vi "WCA_GET_SIS_MODE.vi"(0 "Cartridge Band":u32=10, 1 "Slave Node in":cluster{"Address":i16, "Serial Number":i8[]}={"Address"=19, "Serial Number"=[16, 71, 55, 76, 1, 8, 0, -15]} {"Serial Number" format="%.0x"; "Address" format="%.0x"}, 2 "ObjHandle in":u32, 5 "POL":u32, 7 "sb":u32=1, 11 "error in (no error)":errorcluster) -> (4 "ObjHandle out":u32=92930112, 8 "GET_SIS_MODE":u8, 15 "error out":errorcluster)   [LabVIEW 2017]
uses:
  WCA_Global.vi
panel:
  # "Node Address"
  # "Serial Number"
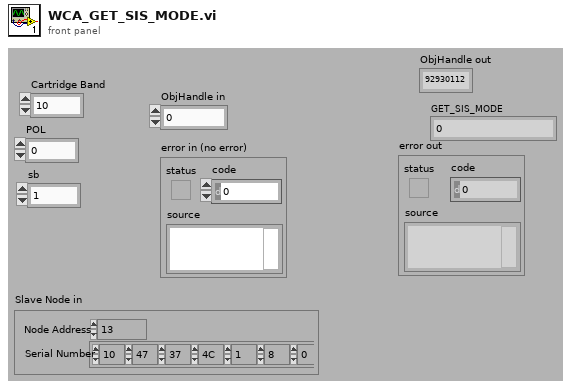
[diagram p1: front panel]
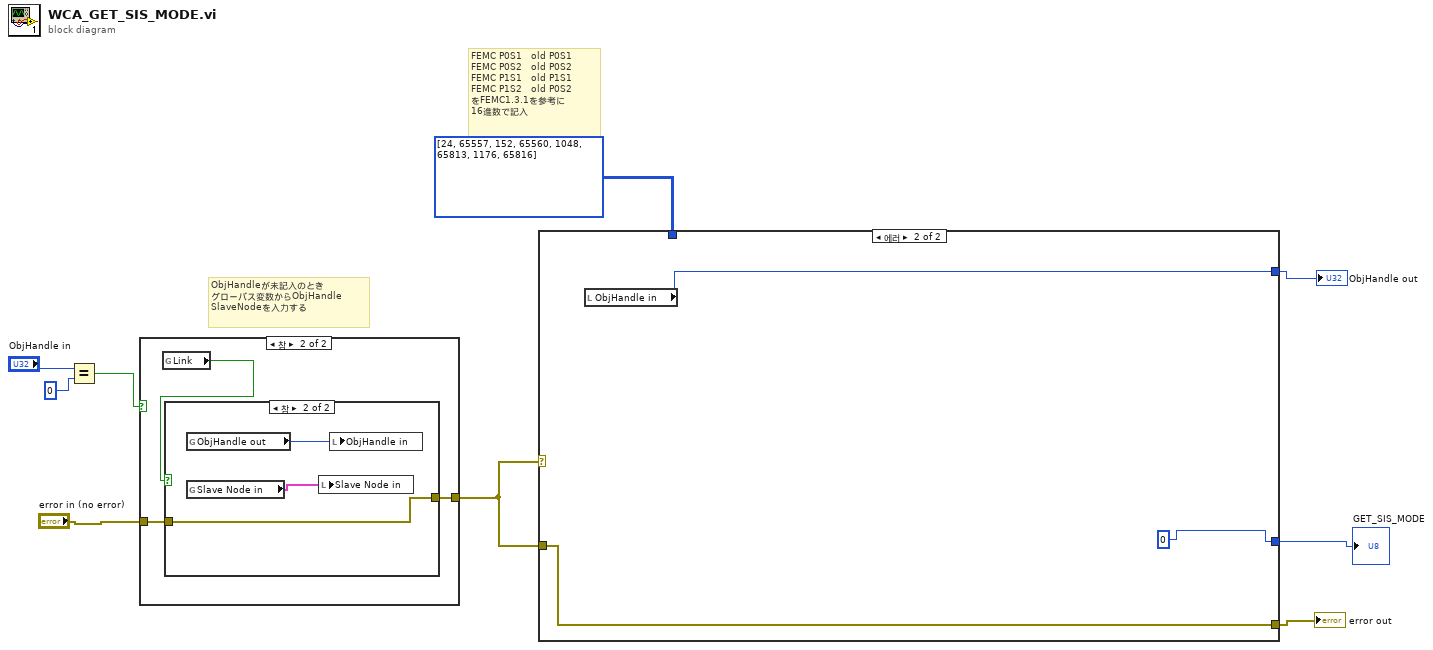
[diagram p0: block diagram]
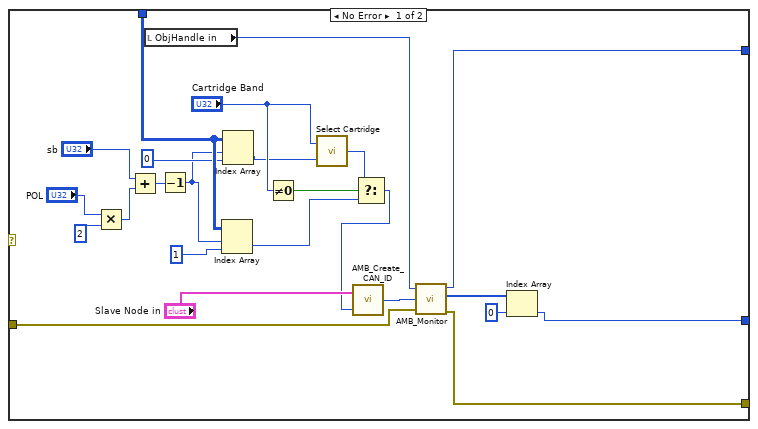
[diagram p2: hidden frame]
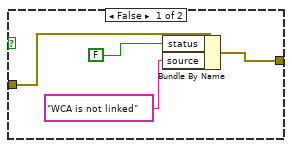
[diagram p4: hidden frame]
diagram:
  # "ObjHandleが未記入のとき\nグローバス変数からObjHandle\nSlaveNodeを入力する"
  # "FEMC P0S1   old P0S1\nFEMC P0S2   old P0S2\nFEMC P1S1   old P1S1\nFEMC P1S2   old P0S2\nをFEMC1.3.1を参考に\n16進数で記入"
  n1 = Equal?(x="ObjHandle in", y=0) -> (x = y?=w7:bool)
  n2 = case shown="참" w7 {
    tunnel: "error in (no error)" -> [w10 w13]
    tunnel: [w10 w12] -> w5
    frame False {
    }
    frame True {
      n3 = global read "WCA_Global.vi" "Link"() -> (w11:bool)
      n4 = case shown="참" w11 {
        tunnel: w13 -> [w17 w18]
        tunnel: [w14 w18] -> w12
        frame False {
          n5 = Bundle By Name(cluster=w17, "status"=FALSE, "source"="WCA is not linked") -> (w14:errorcluster)
        }
        frame True {
          n6 = global read "WCA_Global.vi" "ObjHandle out"() -> (w20:u32)
          n7 = global read "WCA_Global.vi" "Slave Node in"() -> (w19:cluster{"Address":i16, "Serial Number":i8[]})
          n8 = local write "Slave Node in"(w19) -> ()
          n9 = local write "ObjHandle in"(w20) -> ()
        }
      }
    }
  }
  n10 = case shown="에러" w5 {
    tunnel: w5 -> [w23 w47]
    tunnel: [w24 w46] -> w4
    tunnel: [w22 w47] -> w3
    tunnel: i32[][] [[24, 65557], [152, 65560], [1048, 65813], [1176, 65816]] -> [w41 _]
    tunnel: [w21 0] -> w1
    frame No Error {
      n11 = Multiply(x="POL", y=2) -> (x*y=w43:u32)
      n12 = Add(x="sb", y=w43) -> (x+y=w42:u32)
      n13 = local read "ObjHandle in"() -> (w25:u32)
      n14 = Decrement(x=w42) -> (x-1=w34:u32)
      n15 = Index Array(array=w41, index (row)=w34, index (col)=1) -> (element=w37:i32)
      n16 = Index Array(array=w41, index (row)=w34, index (col)=0) -> (element=w36:i32)
      n17 = Not Equal To 0?(x="Cartridge Band") -> (x != 0?=w39:bool)
      n18 = call "Select Cartridge.vi"("Relative Address in"=w36, "Cartridge band"="Cartridge Band") -> ("Relative Address out"=w40:u32)
      n19 = Select(t=w40, s=w39, f=w37) -> (s? t:f=w26:u32)
      n20 = call "AMB_Create_CAN_ID.vi"("Relative Address in"=w26, "Slave Node in"="Slave Node in") -> ("CAN ID out"=w30:u32)
      n21 = call "AMB_Monitor.vi"("ObjHandle in"=w25, "CAN ID in"=w30, "error in"=w23) -> ("ObjHandle out"=w24:u32, "Data Array out"=w29:u8[], "error out"=w22:errorcluster)  [unwired: 1 out]
      n22 = Index Array(array=w29, index=0) -> (element=w21:u8)
    }
    frame Error {
      n23 = local read "ObjHandle in"() -> (w46:u32)
    }
  }
  "ObjHandle out" <- w4
  "error out" <- w3
  "GET_SIS_MODE" <- w1
